vi "Raise Internal Message.vi"(8 "Variant":variant, 9 "Internal Message Type":T1, 10 "error in (no error)":errorcluster, 11 "WAMP Client in":refnum<class "WAMP Client.lvclass">) -> (2 "error out":errorcluster, 3 "WAMP Client out":refnum<class "WAMP Client.lvclass">)   [LabVIEW 2020, in "wamplv.lvlib" / "WAMP Client.lvclass"]
uses:
  WAMP Client.lvclass
  TypeDef/Internal Message Type.ctl
  WAMP Client.lvclass/WAMP Client.ctl
  TypeDef/Internal Message.ctl
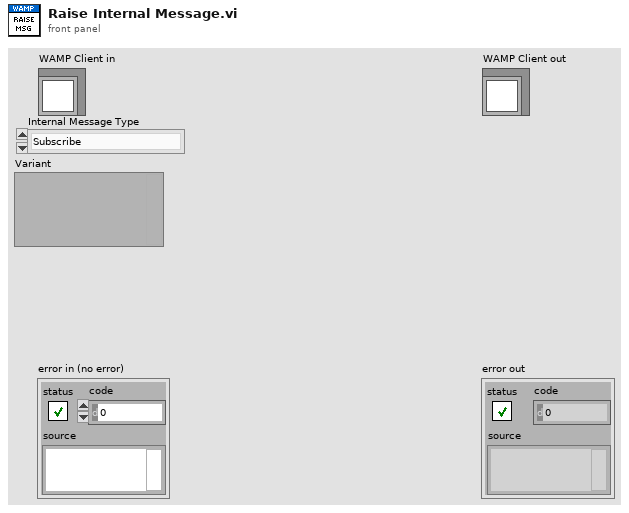
[diagram p1: front panel]
types:
  T1 = typedef "wamplv.lvlib/WAMP Client.lvclass/Internal Message Type.ctl" = enum16{"Subscribe", "Handle Subscribed", "Handle Event", "Unsubscribe", "Handle Unsubscribed", "Publish", "Handled Published", "Goodbye", "Handle Goodbye", "Call", "Handle Result", "Register", "Handle Registered", "Unregister", "Handle Unregistered", "Handle Invocation", "Yield", "Error"}
  T2 = typedef "wamplv.lvlib/WAMP Client.lvclass/Internal Message.ctl" = cluster{"Internal Message Type":T1, "Variant":variant}
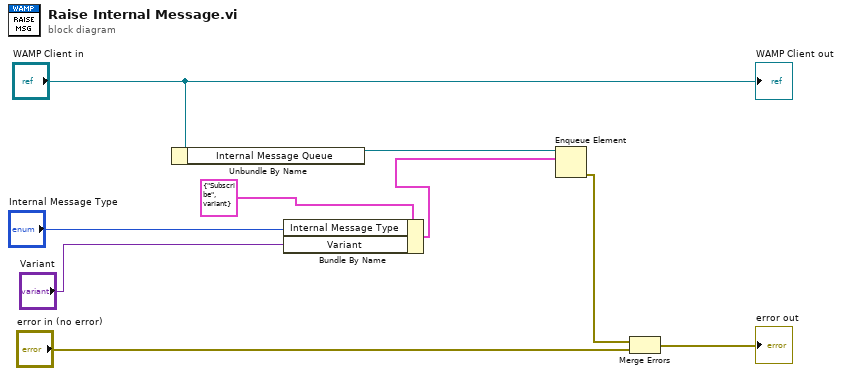
[diagram p0: block diagram]
diagram:
  n1 = Unbundle By Name("WAMP Client in") -> ("Internal Message Queue"=w6:refnum<queue>)
  n2 = Bundle By Name(cluster=T2 {"Internal Message Type"=enum."Subscribe", "Variant"=variant} ("Cluster"), "Internal Message Type"="Internal Message Type", "Variant"="Variant") -> (w5:T2)
  n3 = Enqueue Element(queue=w6, element=w5) -> (error out=w2:errorcluster)  [unwired: 2 in, 2 out]
  n4 = Merge Errors(w2, "error in (no error)") -> (→"error out":errorcluster)
  "WAMP Client out" <- "WAMP Client in"
